vi "Get Creator Alias.vi"(11 "Base Addresses Strategy in":refnum<class "Base Addresses Strategy.lvclass">) -> (2 "Creator Alias":string)   [LabVIEW 2021, in "jettl.lvlib" / "Addresses Strategy.lvlib" / "Base Addresses Strategy.lvclass"]
uses:
  Base Addresses Strategy.lvclass
  Base Addresses Strategy.lvclass/Base Addresses Strategy.ctl
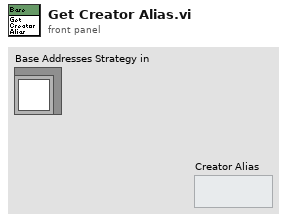
[diagram p1: front panel]
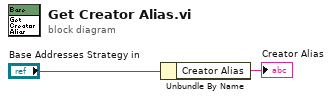
[diagram p0: block diagram]
diagram:
  n1 = Unbundle By Name("Base Addresses Strategy in") -> ("Creator Alias"=→"Creator Alias":string)
